vi "Update List of Controls Tree.vi"(8 "error in (no error)":errorcluster, 11 "Data Cluster":T1) -> (0 "error out":errorcluster, 3 "Items":T6(array[cluster]))   [LabVIEW 2021, in "Control Property Tree.lvlib"]
uses:
  Control Property Tree.lvlib
  Module Data--cluster.ctl
  Ctrl Properties Map Data.ctl
  Property array.ctl
  Selected Ctrls - List of Controls.ctl
  Selected Ctrls - List of Properties.ctl
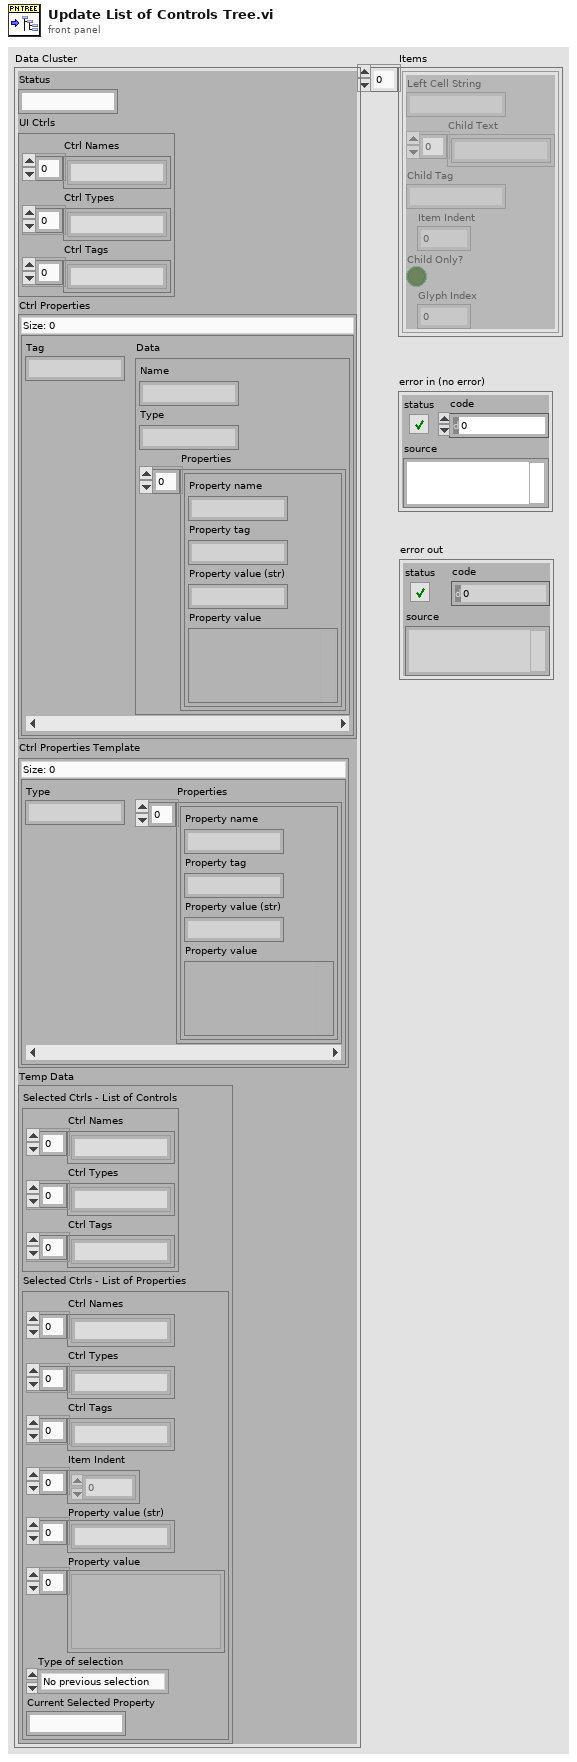
[diagram p1: front panel]
types:
  T1 = typedef "Control Property Tree.lvlib/Module Data--cluster.ctl" = cluster{"Status":string, "UI Ctrls":cluster{"Ctrl Names":string[], "Ctrl Types":string[], "Ctrl Tags":string[]}, "Ctrl Properties":map{string, T2}, "Ctrl Properties Template":map{string, T3}, "Temp Data":cluster{"Selected Ctrls - List of Controls":T4, "Selected Ctrls - List of Properties":T5}}
  T2 = typedef "Control Property Tree.lvlib/Ctrl Properties Map Data.ctl" = cluster{"Name":string, "Type":string, "Properties":T3}
  T3 = typedef "Control Property Tree.lvlib/Property array.ctl" = cluster{"Property name":string, "Property tag":string, "Property value (str)":string, "Property value":variant}[]
  T4 = typedef "Control Property Tree.lvlib/Selected Ctrls - List of Controls.ctl" = cluster{"Ctrl Names":string[], "Ctrl Types":string[], "Ctrl Tags":string[]}
  T5 = typedef "Control Property Tree.lvlib/Selected Ctrls - List of Properties.ctl" = cluster{"Ctrl Names":string[], "Ctrl Types":string[], "Ctrl Tags":string[], "Item Indent":i32[], "Property value (str)":string[], "Property value":variant[], "Type of selection":enum16{"No previous selection", "Control selected", "Property selected"}, "Current Selected Property":string}
  T6 = cluster{"Left Cell String":string, "Child Text":string[], "Child Tag":string, "Item Indent":i32, "Child Only?":bool, "Glyph Index":i32}[]
  T7 = cluster{"Left Cell String":string, "Child Text":string[], "Child Tag":string, "Item Indent":i32, "Child Only?":bool, "Glyph Index":i32}
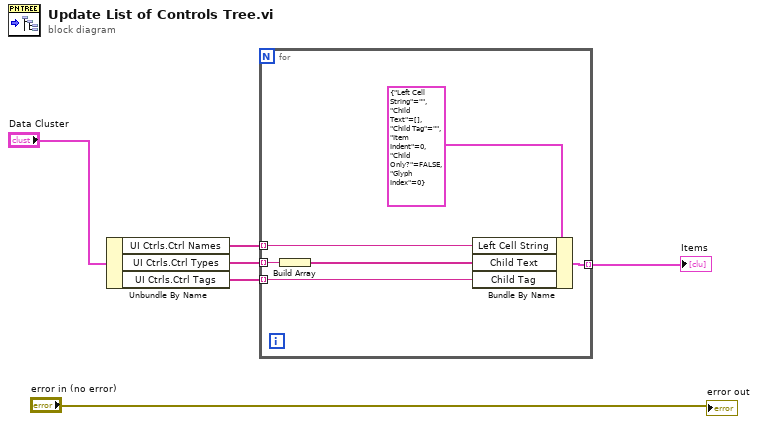
[diagram p0: block diagram]
diagram:
  n1 = Unbundle By Name("Data Cluster") -> ("UI Ctrls.Ctrl Names"=w3:string[], "UI Ctrls.Ctrl Types"=w4:string[], "UI Ctrls.Ctrl Tags"=w5:string[])
  n2 = for {
    tunnel: w3 -> [w10] mode=indexing
    tunnel: w4 -> [w9] mode=indexing
    tunnel: w5 -> [w7] mode=indexing
    tunnel: [w12] -> w6 mode=indexing
    n3 = Build Array(w9) -> (w8:string[])
    n4 = Bundle By Name(cluster=T7 {"Left Cell String"="", "Child Text"=[], "Child Tag"="", "Item Indent"=0, "Child Only?"=FALSE, "Glyph Index"=0} ("Item"), "Left Cell String"=w10, "Child Text"=w8, "Child Tag"=w7) -> (w12:T7)
  }
  "Items" <- w6
  "error out" <- "error in (no error)"
